vi "Untitled 2.vi"() -> ()   [LabVIEW 2017]
panel:
  in  "vi path":path
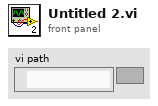
[diagram p1: front panel]
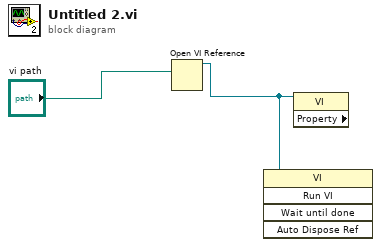
[diagram p0: block diagram]
diagram:
  n1 = Open VI Reference(vi path="vi path") -> (vi reference=w1:refnum<vi>)  [unwired: 5 in, 1 out]
  n2 = invoke class="VI" method="Run VI"(reference=w1) -> ()  [unwired: 4 in, 5 out]
  n3 = property class="VI" props=[](reference=w1) -> ()  [unwired: 1 in, 3 out]
